vi "MultiJoint анимация.vi"() -> ()   [LabVIEW 2020]
panel:
  in  "Shoulder Size 2":dbl
  in  "Shoulder Size":dbl
  in  "4 joint":dbl(slide) scale=0.0..180.0
  in  "3 joint":dbl(slide) scale=0.0..180.0
  in  "2 joint":dbl(slide) scale=0.0..180.0
  in  "1 joint":dbl(slide) scale=0.0..180.0
  out "XY Graph":cluster{dbl[], dbl[]}(graph)
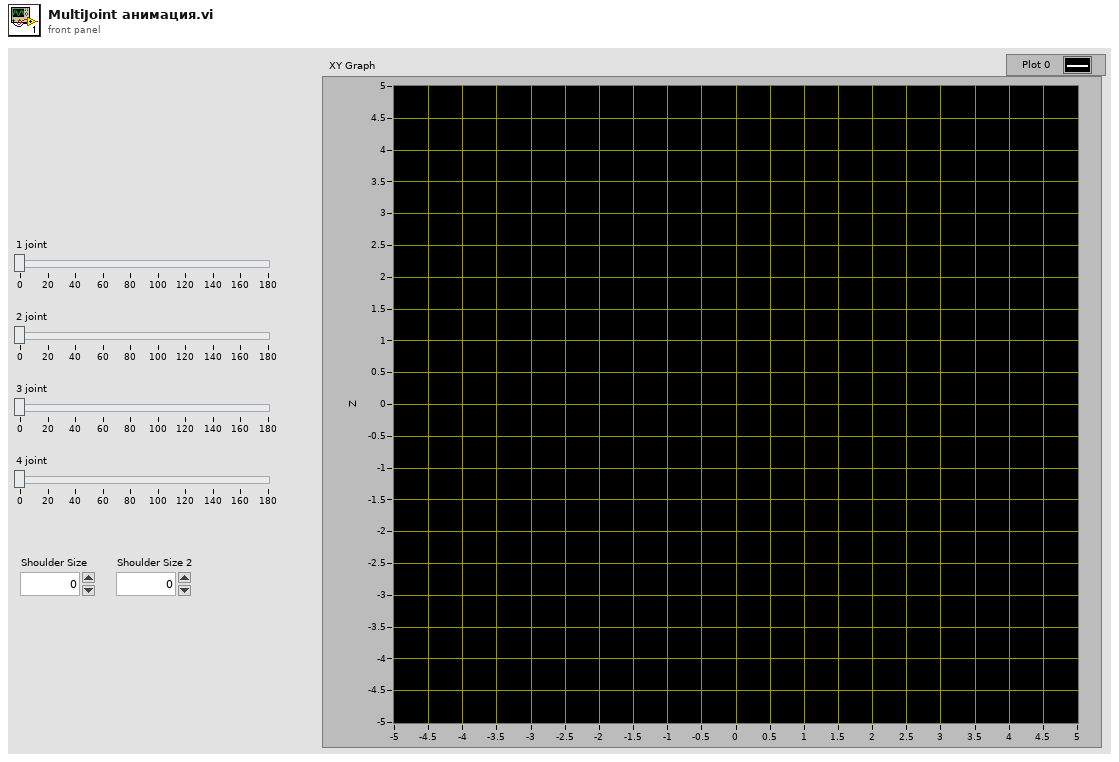
[diagram p1: front panel]
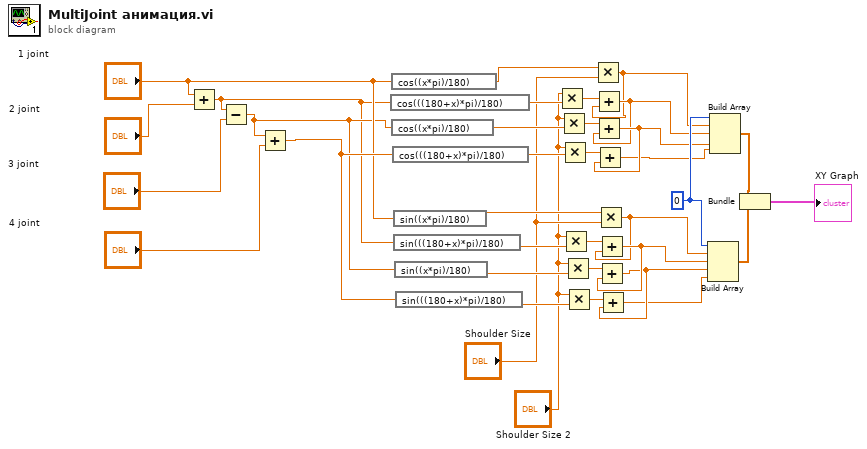
[diagram p0: block diagram]
diagram:
  w30 = 0
  n1 = Add(x="1 joint", y="2 joint") -> (x+y=w20:dbl)
  n2 = Subtract(x=w20, y="3 joint") -> (x-y=w21:dbl)
  n3 = Add(x=w21, y="4 joint") -> (x+y=w23:dbl)
  n4 = expression code="cos(((180+x)*pi)/180)"(w20) -> (w16:dbl)
  n5 = expression code="cos((x*pi)/180)"("1 joint") -> (w32:dbl)
  n6 = expression code="cos((x*pi)/180)"(w21) -> (w11:dbl)
  n7 = expression code="cos(((180+x)*pi)/180)"(w23) -> (w12:dbl)
  n8 = expression code="sin((x*pi)/180)"("1 joint") -> (w31:dbl)
  n9 = expression code="sin(((180+x)*pi)/180)"(w20) -> (w14:dbl)
  n10 = expression code="sin((x*pi)/180)"(w21) -> (w7:dbl)
  n11 = expression code="sin(((180+x)*pi)/180)"(w23) -> (w6:dbl)
  n12 = Multiply(x="Shoulder Size 2", y=w16) -> (x*y=w17:dbl)
  n13 = Multiply(x="Shoulder Size 2", y=w11) -> (x*y=w13:dbl)
  n14 = Multiply(x="Shoulder Size 2", y=w12) -> (x*y=w10:dbl)
  n15 = Multiply(x="Shoulder Size 2", y=w14) -> (x*y=w15:dbl)
  n16 = Multiply(x="Shoulder Size 2", y=w7) -> (x*y=w8:dbl)
  n17 = Multiply(x="Shoulder Size 2", y=w6) -> (x*y=w9:dbl)
  n18 = Multiply(x=w32, y="Shoulder Size") -> (x*y=w19:dbl)
  n19 = Add(x=w17, y=w19) -> (x+y=w28:dbl)
  n20 = Add(x=w13, y=w28) -> (x+y=w29:dbl)
  n21 = Add(x=w10, y=w29) -> (x+y=w27:dbl)
  n22 = Multiply(x=w31, y="Shoulder Size") -> (x*y=w18:dbl)
  n23 = Add(x=w15, y=w18) -> (x+y=w26:dbl)
  n24 = Add(x=w8, y=w26) -> (x+y=w25:dbl)
  n25 = Add(x=w9, y=w25) -> (x+y=w24:dbl)
  n26 = Build Array(w30, w18, w26, w25, w24) -> (w33:dbl[])
  n27 = Build Array(w30, w19, w28, w29, w27) -> (w34:dbl[])
  n28 = Bundle(w34, w33) -> (→"XY Graph":cluster{dbl[], dbl[]})  [unwired: 1 in]
